vi "Support guidePanel.vi"() -> ()   [LabVIEW 2018]
uses:
  PublicSubVI/Class/DataXML/DataXML.lvclass
  <vilib>/Utility/sysdir.llb/System Directory Type.ctl
  PublicSubVI/Class/DataXML/DataXML dataType.ctl
panel:
  out "appended path":path
  in  "ESI":bool
  in  "MALDI":bool
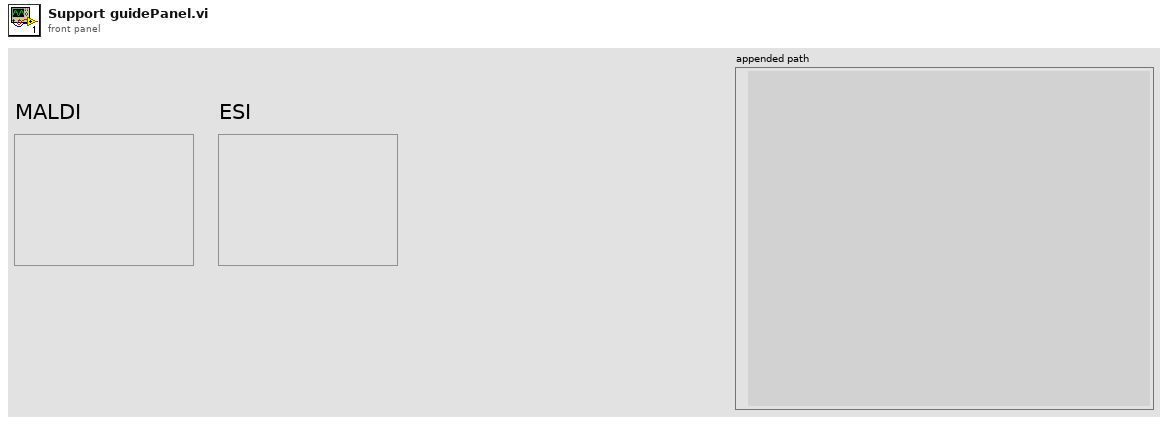
[diagram p1: front panel]
types:
  T1 = typedef "DataXML dataType.ctl" = enum16{"Instrument", "UserInterface", "SampleType", "UserDefined"}
  T2 = typedef "System Directory Type.ctl" = i32
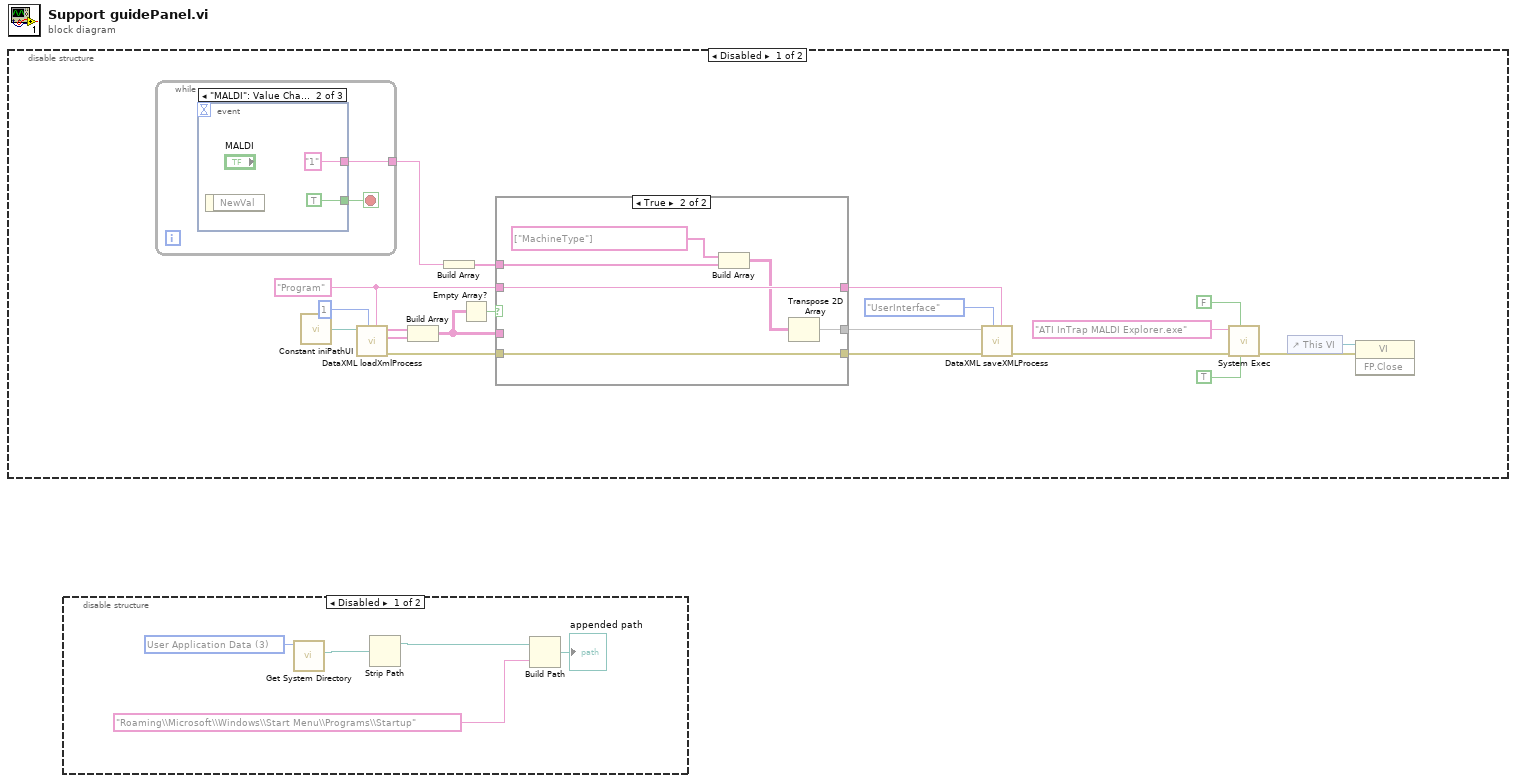
[diagram p0: block diagram]
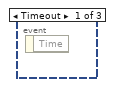
[diagram p3: hidden frame]
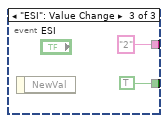
[diagram p4: hidden frame]
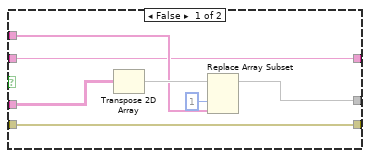
[diagram p5: hidden frame]
diagram:
  n1 = disable-structure shown="Disabled" {
    frame Disabled {
      w17 = "Program" ("target name")
      n2 = while {
        tunnel: [w21] -> w14
        stop <- w22 stop-if-true
        n3 = event shown="[1] \"MALDI\": Value Change" {
          selector: _ -> [_ _ _]
          dyn-events: _ -> [_ _ _]
          timeout: _ -> [_ _ _]
          tunnel: [_ TRUE TRUE] -> w22
          tunnel: [_ "1" "2"] -> w21
          event Timeout {
            n4 = event-data() -> ()  [unwired: 1 in, 1 out]
          }
          event "MALDI": Value Change {
            n5 = event-data() -> ()  [unwired: 1 in, 1 out]
          }
          event "ESI": Value Change {
            n6 = event-data() -> ()  [unwired: 1 in, 1 out]
          }
        }
      }
      n7 = call "Constant iniPathUI.vi"() -> ("appended path"=w4:path)
      n8 = call "DataXML loadXmlProcess.vi"("target name"=w17, "level"=u8 1, "xml_data_path"=w4) -> ("error IO"=w7:errorcluster, "value"=w18:string[], "name"=w19:string[])  [unwired: 5 in, 1 out]
      n9 = Build Array(w19, w18) -> (w16:string[][])
      n10 = Build Array(w14) -> (w13:string[])
      n11 = Empty Array?(array=w16) -> (empty?=w15:bool)
      n12 = case shown="True" w15 {
        tunnel: w16 -> [w33 _]
        tunnel: w17 -> [w28 w37]
        tunnel: w13 -> [w30 w38]
        tunnel: [w29 w34] -> w3
        tunnel: [w28 w37] -> w2
        tunnel: w7 -> [w27 w36]
        tunnel: [w27 w36] -> w6
        frame False {
          n13 = Transpose 2D Array(2D array=w33) -> (transposed array=w32:string[][])
          n14 = Replace Array Subset(array=w32, new element=w30, index (col)=1 ("disabled index (col)")) -> (w29:string[][])  [unwired: 1 in]
        }
        frame True {
          n15 = Build Array(string[] ["MachineType"], w38) -> (w35:string[][])
          n16 = Transpose 2D Array(2D array=w35) -> (transposed array=w34:string[][])
        }
      }
      n17 = call "DataXML saveXMLProcess.vi"("addTagName"=w2, "dataType"=DataXML_dataType."UserInterface", "error in (no error)"=w6, "newData"=w3) -> ("error out"=w5:errorcluster)  [unwired: 7 in]
      n18 = call <vilib>:"System Exec.vi"("run minimized? (F)"=TRUE, "wait until completion? (T)"=FALSE, "error in (no error)"=w5, "command line"="ATI InTrap MALDI Explorer.exe") -> ("error out"=w8:errorcluster)  [unwired: 4 in, 3 out]
      n19 = control-ref of="This VI"() -> (w9:refnum<vi>)
      n20 = invoke class="VI" method="FP.Close"(reference=w9, error in=w8) -> ()  [unwired: 1 in, 3 out]
    }
    frame Enabled {
    }
  }
  n21 = disable-structure shown="Disabled" {
    frame Disabled {
      w44 = T2 3 items=["User Home"=0, "User Desktop"=1, "User Documents"=2, "User Application Data"=3, "User Preferences"=4, "User Temporary"=5, "Public Documents"=6, "Public Application Data"=7, "Public Preferences"=8, "Public Cache"=13, "System Core Libraries"=9, "System Installed Libraries"=10, "Application Files"=11, "Boot Volume Root"=12] ("system directory type")
      n22 = call <vilib>:"Get System Directory.vi"("system directory type"=w44) -> ("system directory"=w43:path)  [unwired: 10 in]
      n23 = Strip Path(path=w43) -> (stripped path=w42:path)  [unwired: 1 out]
      n24 = Build Path(base path=w42, name or relative path="Roaming\\Microsoft\\Windows\\Start Menu\\Programs\\Startup") -> (appended path=→"appended path":path)
    }
    frame Enabled {
    }
  }
